vi "Humidity Updated.vi"(8 "error in":errorcluster, 11 "Humidity":dbl) -> (0 "error out":errorcluster)   [LabVIEW 2026, in "Servo Motor Emulator.lvlib"]
doc: "_____\nCreated using DQMH Framework: Event Scripter 7.1.2.1547."
uses:
  Servo Motor Emulator.lvlib
  Humidity Updated Argument--cluster.ctl
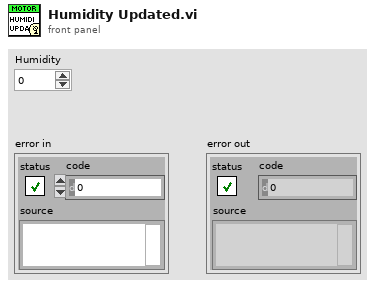
[diagram p1: front panel]
types:
  T1 = typedef "Servo Motor Emulator.lvlib/Humidity Updated Argument--cluster.ctl" = cluster{"Humidity":dbl}
  T2 = typedef "Servo Motor Emulator.lvlib/Broadcast Events--cluster.ctl" = cluster{"Module Did Init":refnum<user-event>, "Status Updated":refnum<user-event>, "Error Reported":refnum<user-event>, "Module Did Stop":refnum<user-event>, "Update Module Execution Status":refnum<user-event>, "Temperature Updated":refnum<user-event>, "Humidity Updated":refnum<user-event>}
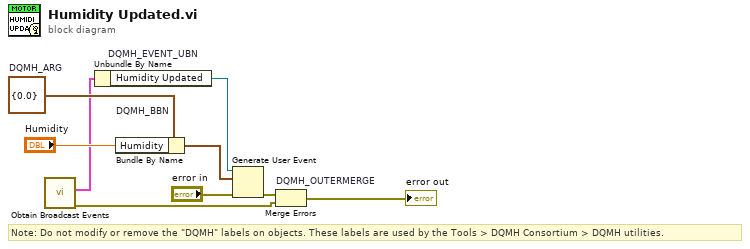
[diagram p0: block diagram]
diagram:
  w4 = T1 {"Humidity"=0.0}  # DQMH_ARG
  # "Note: Do not modify or remove the \"DQMH\" labels on objects. These labels are used by the Tools > DQMH Consortium > DQMH utilities."
  n1 = call "Obtain Broadcast Events.vi"() -> ("error out"=w2:errorcluster, "Servo Motor Emulator Broadcast Events"=w1:T2)  [unwired: 10 in]
  n2 = Unbundle By Name "DQMH_EVENT_UBN"(w1) -> ("Humidity Updated"=w6:refnum<user-event>)
  n3 = Bundle By Name "DQMH_BBN"(cluster=w4, "Humidity"="Humidity") -> (w7:T1)
  n4 = Generate User Event(user event=w6, event data cluster=w7, error in="error in") -> (error out=w5:errorcluster)  [unwired: 1 in, 1 out]
  n5 = Merge Errors "DQMH_OUTERMERGE"(w5, w2) -> (→"error out":errorcluster)
